vi "Control Intake Reverse.vi"(11 "Avoid Race Condition":bool) -> ()   [LabVIEW 2020]
uses:
  Framework/Robot Global Data.vi
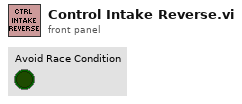
[diagram p1: front panel]
types:
  T1 = typedef "Command Status Info.ctl" = cluster{"Name":string, "Status":T2, "notifier out":T3}
  T2 = typedef "Completion Status.ctl" = enum16{"Successful", "Aborted", "Incomplete"}
  T3 = typedef "Completion Notifier.ctl" = refnum<notifier>
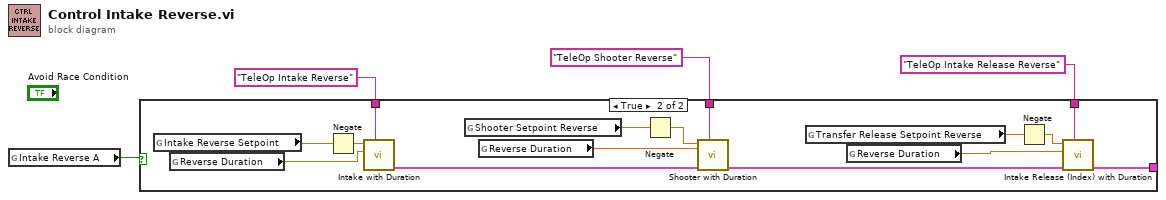
[diagram p0: block diagram]
diagram:
  n1 = global read "Robot Global Data.vi" "Intake Reverse A"() -> (w4:bool)
  n2 = case shown="True" w4 {
    tunnel: "TeleOp Intake Reverse" ("Description") -> [_ w19]
    tunnel: "TeleOp Shooter Reverse" ("Description") -> [_ w14]
    tunnel: "TeleOp Intake Release Reverse" ("Description") -> [_ w13]
    tunnel: [_ w10] -> _
    frame False {
    }
    frame True {
      n3 = global read "Robot Global Data.vi" "Intake Reverse Setpoint"() -> (w17:dbl)
      n4 = global read "Robot Global Data.vi" "Reverse Duration"() -> (w16:dbl)
      n5 = Negate(x=w17) -> (-x=w18:dbl)
      n6 = call "Intake with Duration.vi"("Description"=w19, "Duration (s)"=w16, "Setpoint"=w18) -> ("Command Info Out"=w11:T1)  [unwired: 8 in]
      n7 = global read "Robot Global Data.vi" "Shooter Setpoint Reverse"() -> (w9:dbl)
      n8 = global read "Robot Global Data.vi" "Reverse Duration"() -> (w8:dbl)
      n9 = Negate(x=w9) -> (-x=w6:dbl)
      n10 = call "Shooter with Duration .vi"("Description"=w14, "Command Info In"=w11, "Duration (s)"=w8, "Setpoint"=w6) -> ("Command Info Out"=w12:T1)  [unwired: 7 in]
      n11 = global read "Robot Global Data.vi" "Transfer Release Setpoint Reverse"() -> (w7:dbl)
      n12 = global read "Robot Global Data.vi" "Reverse Duration"() -> (w15:dbl)
      n13 = Negate(x=w7) -> (-x=w5:dbl)
      n14 = call "Intake Release (Index) with Duration.vi"("Description"=w13, "Command Info In"=w12, "Duration (s)"=w15, "Setpoint"=w5) -> ("Command Info Out"=w10:T1)  [unwired: 7 in]
    }
  }
